vi "VCS Read Channel Vector Size.vi"(8 "error in (no error)":errorcluster, 11 "axis in":cluster{"keyHandle":u32, "nodeId":u16}={"keyHandle"=0, "nodeId"=1}) -> (0 "error out":errorcluster, 1 "vector size":u32, 3 "axis out":cluster{"keyHandle":u32, "nodeId":u16}={"keyHandle"=0, "nodeId"=1})   [LabVIEW 2019, in "maxonEPOS.lvlib"]
doc: "<B>VCS_ReadChannelVectorSize</B> returns the maximal number of samples per variable. This parameter is dynamically calculated by the data recorder."
uses:
  Examples/maxonEPOS.lvlib
  Resources/EposCmd.dll
  Resources/EposCmd64.dll
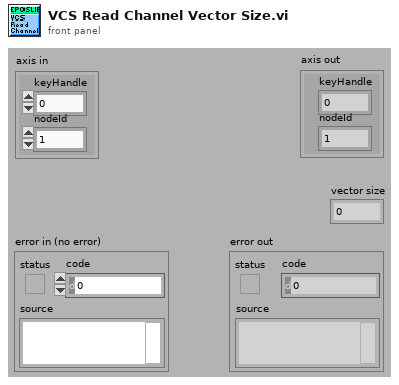
[diagram p1: front panel]
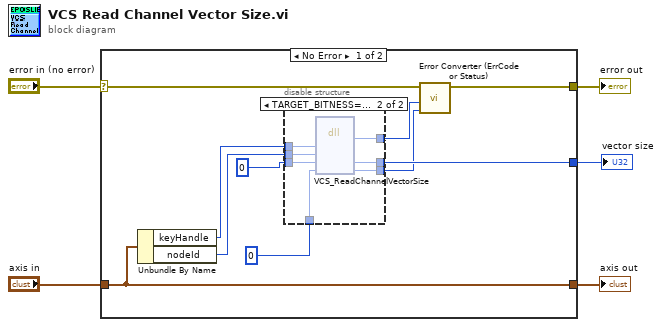
[diagram p0: block diagram]
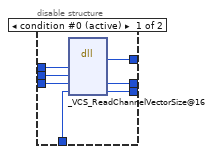
[diagram p2: hidden frame]
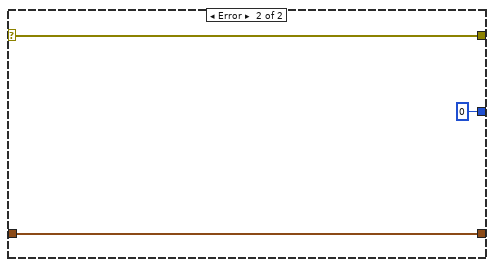
[diagram p3: hidden frame]
diagram:
  n1 = case shown="No Error" "error in (no error)" {
    selector: "error in (no error)" -> [w13 w31]
    tunnel: "axis in" -> [w15 w32]
    tunnel: [w15 w32] -> w4
    tunnel: [w14 w31] -> w3
    tunnel: [w12 u32 0 ("pVectorSize")] -> w1
    frame No Error {
      n2 = Unbundle By Name(w15) -> ("keyHandle"=w9:u32, "nodeId"=w8:u16)
      n3 = disable-structure shown="TARGET_BITNESS==64" {
        disable-tunnel: [w22 w29] -> w12
        disable-tunnel: [w21 w28] -> w11
        disable-tunnel: [w20 w27] -> w10
        disable-tunnel: w9 -> [w19 w26]
        disable-tunnel: w8 -> [w18 w25]
        disable-tunnel: u32 0 ("pErrorCode") -> [w17 w24]
        disable-tunnel: u32 0 ("pVectorSize") -> [w16 w23]
        frame condition #0 (active) {
          n4 = dll-call lib="C:/workspace/project/scancon/sw/SSI_Tool/InstrumentsInterfaces/Motordriver/maxon EPOS/Resources/EposCmd.*" fn="_VCS_ReadChannelVectorSize@16" ("VCS_ReadChannelVectorSize")("KeyHandle"=w19, "NodeId"=w18, "pVectorSize"=w16, "pErrorCode"=w17) -> (w20:i32, "pVectorSize"=w22:u32, "pErrorCode"=w21:u32)  [unwired: 5 in, 2 out]
        }
        frame condition #1 {
          n5 = dll-call lib="C:/Sources/LabView/maxon EPOS/Resources/EposCmd64.dll" fn="VCS_ReadChannelVectorSize"("KeyHandle"=w26, "NodeId"=w25, "pVectorSize"=w23, "pErrorCode"=w24) -> ("Rückgabetyp"=w27:i32, "pVectorSize"=w29:u32, "pErrorCode"=w28:u32)  [unwired: 5 in, 2 out]
        }
      }
      n6 = call "Error Converter (ErrCode or Status).vi"("error code"=w11, "return type"=w10, "error in (no error)"=w13) -> ("error out"=w14:errorcluster)  [unwired: 7 in]
    }
    frame Error {
    }
  }
  "vector size" <- w1
  "error out" <- w3
  "axis out" <- w4
